vi "Alarm & Event List.vi"(8 "error in (no error)":errorcluster, 10 "Subview Stop Event":refnum<user-event>, 11 "Subsystem URL":refnum<k21>="\\\\localhost\\ABCDEFG\\TCU3") -> ()   [LabVIEW 2024]
doc: "Displays the current alarms and events for the specified subsystem. This VI is a subview of the Detailed View."
uses:
  Controls/Client/Alarm Description Item.ctl
  Controls/Client/Alarm & Event List - Data.ctl
  Controls/Client/Initialization Status.ctl
  <vilib>/lvdsc/alarm/Acknowledge Alarms By Instance.vi
  Shared/User Event - Stop.lvlib
  <vilib>/lvdsc/NI_DSC.lvlib
panel:
  out "error out":errorcluster
  in  "Acknowledge All":bool
  in  "Acknowledge":bool
  in  "Alarm Summary":i32(listbox)
  in  "Alarm Display Format":T1[](array[typedef])=[enum."alarm URL", enum."event?", enum."value", enum."set time", enum."ack time"]
  in  "Stop":bool
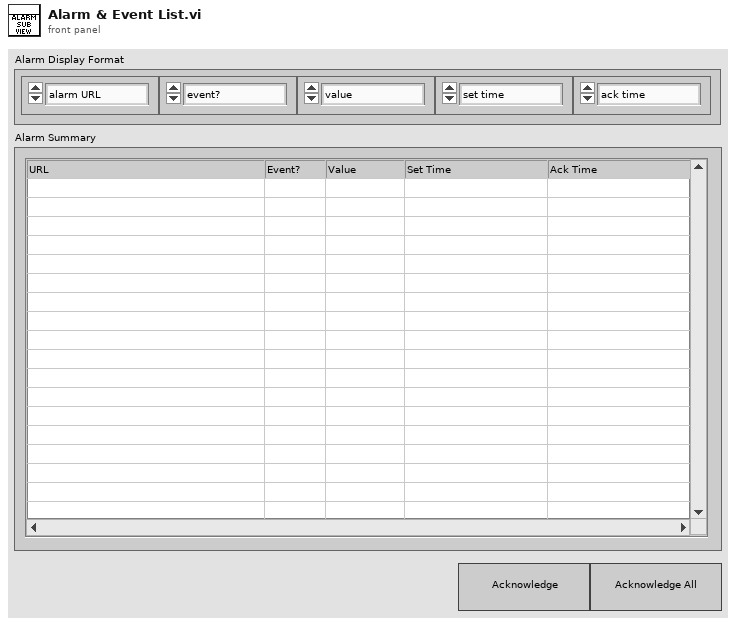
[diagram p1: front panel]
types:
  T1 = typedef "Alarm Description Item.ctl" = enum16{"alarm URL", "event?", "set time", "ack time", "clear time", "set user", "ack user", "clear user", "set point", "value", "priority", "alarm area", "alarm description", "ack comment"}
  T2 = typedef "Alarm & Event List - Data.ctl" = cluster{"Subsystem URL":refnum<k21>, "Variables":refnum<k21>[], "Subview Stop Event":refnum<user-event>, "Alarm & Event Notifications":refnum<user-event>, "Initialization Status":T3, "Value List Reference":refnum<vi>, "Alarms":cluster{"alarm URL":string, "set time":timestamp, "set user":string, "ack time":timestamp, "ack user":string, "clear time":timestamp, "clear user":string, "setpoint":enum16{""}, "value":dbl, "priority":u32, "alarm area":string, "alarm description":string, "ack comment":string, "event?":bool, "Refnum":u64}[]}
  T3 = typedef "Initialization Status.ctl" = enum16{"Initializing", "Initialized"}
  T4 = cluster{"alarm URL":string, "set time":timestamp, "set user":string, "ack time":timestamp, "ack user":string, "clear time":timestamp, "clear user":string, "setpoint":enum16{""}, "value":dbl, "priority":u32, "alarm area":string, "alarm description":string, "ack comment":string, "event?":bool, "Refnum":u64}
  T5 = cluster{"alarm URL":string, "set time":timestamp, "set user":string, "ack time":timestamp, "ack user":string, "clear time":timestamp, "clear user":string, "setpoint":enum16{""}, "value":dbl, "priority":u32, "alarm area":string, "alarm description":string, "ack comment":string, "event?":bool, "Refnum":u64}[]
  T6 = cluster{"alarm URL":string, "set time":timestamp, "set user":string, "ack time":timestamp, "ack user":string, "clear time":timestamp, "clear user":string, "setpoint":dbl, "value":dbl, "priority":u32, "alarm area":string, "alarm description":string, "ack comment":string, "event?":bool, "Refnum":u64}[]
  T7 = cluster{"# active alarms occurrences":i32, "any alarm occurrences?":bool, "# unack alarms occurrences":i32, "any unack alarm occurrences?":bool, "# shared variables with active alarms":i32, "any shared variables with alarms?":bool, "# shared variables with unack alarms":i32, "any shared variables with unack alarms?":bool}
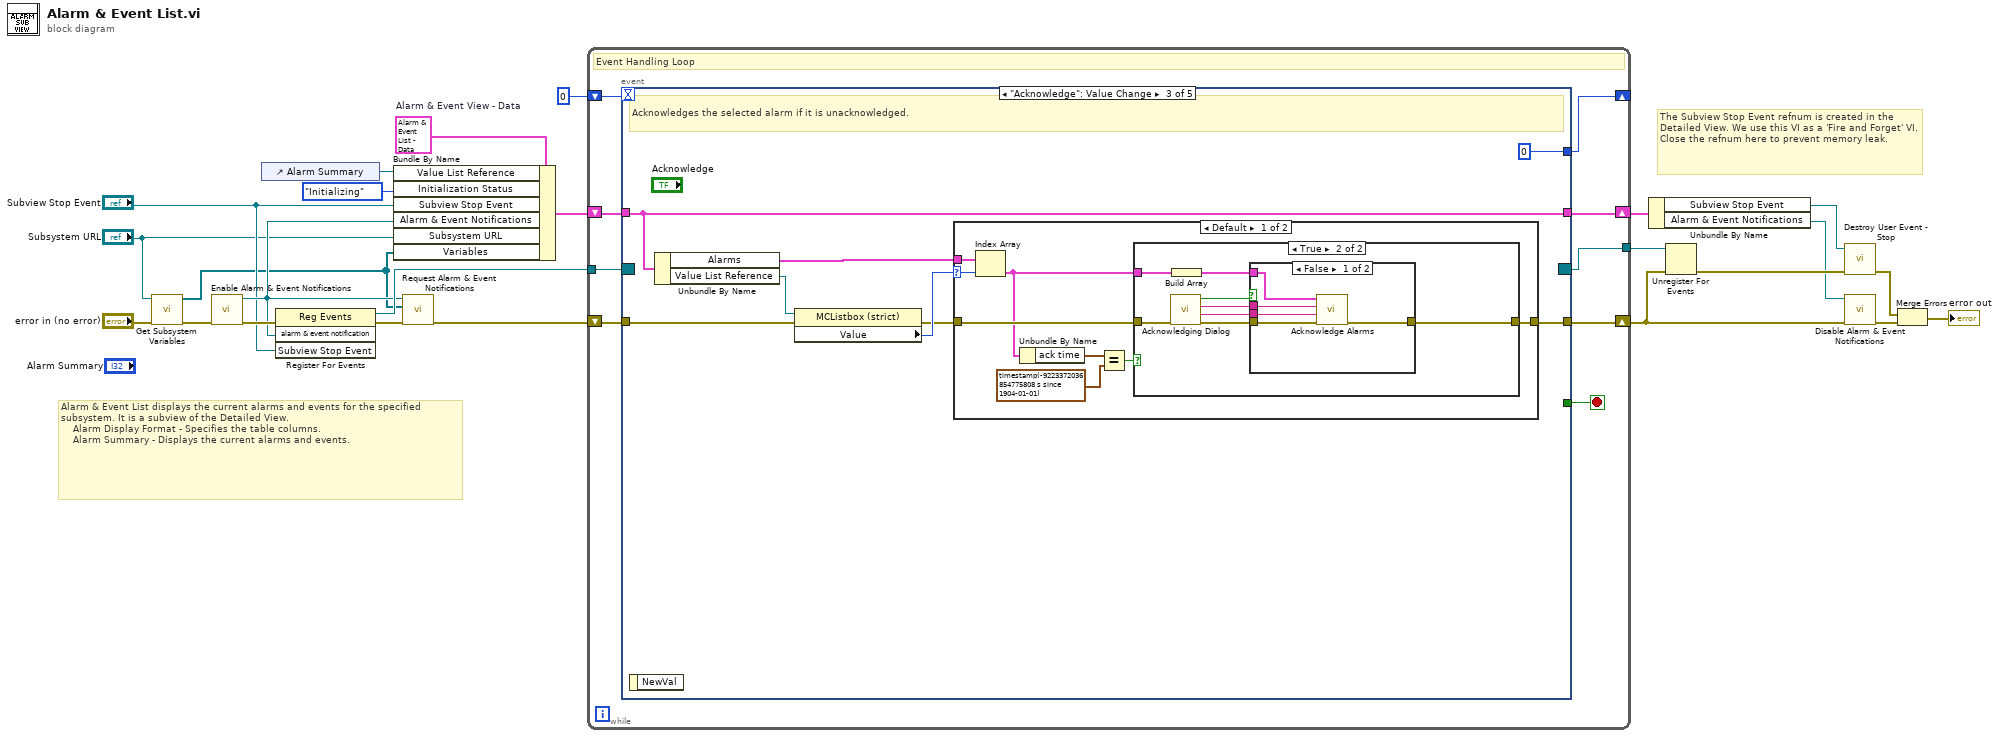
[diagram p0: block diagram]
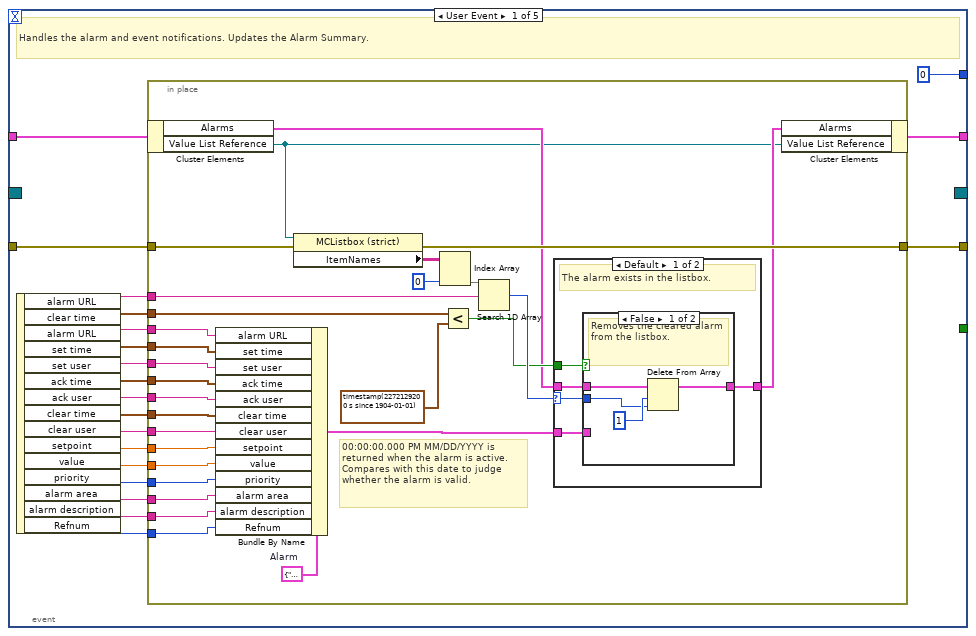
[diagram p2: hidden frame]
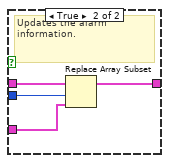
[diagram p3: hidden frame]
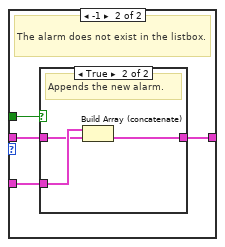
[diagram p4: hidden frame]
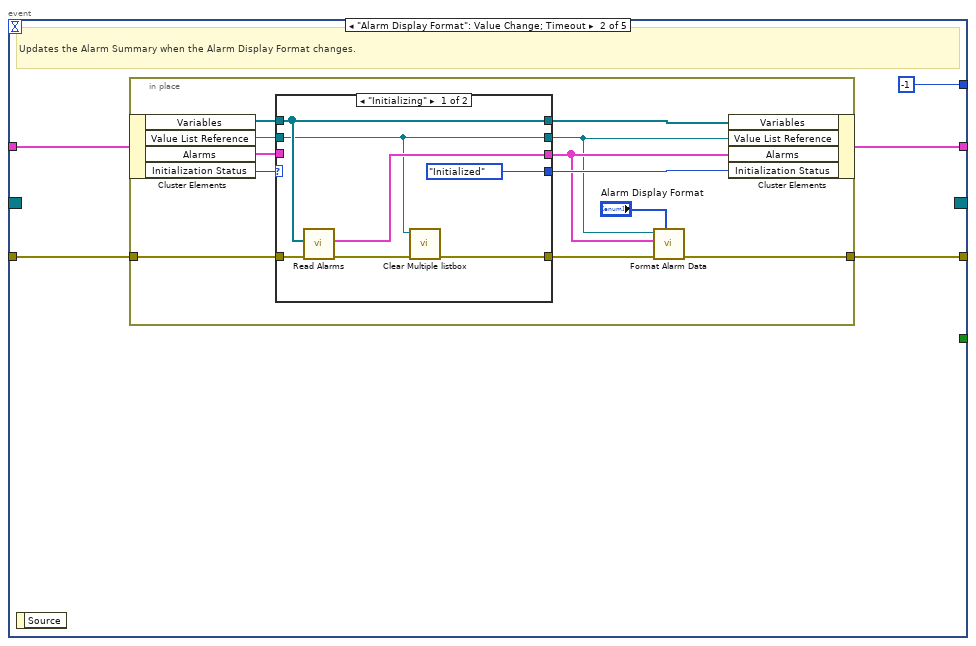
[diagram p6: hidden frame]
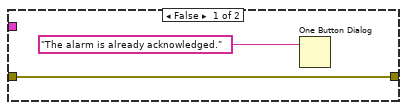
[diagram p8: hidden frame]
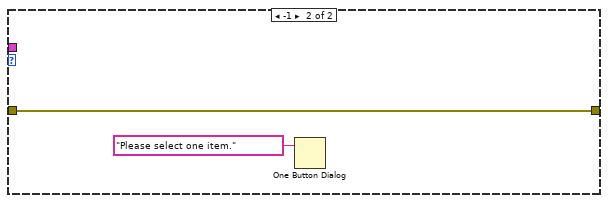
[diagram p10: hidden frame]
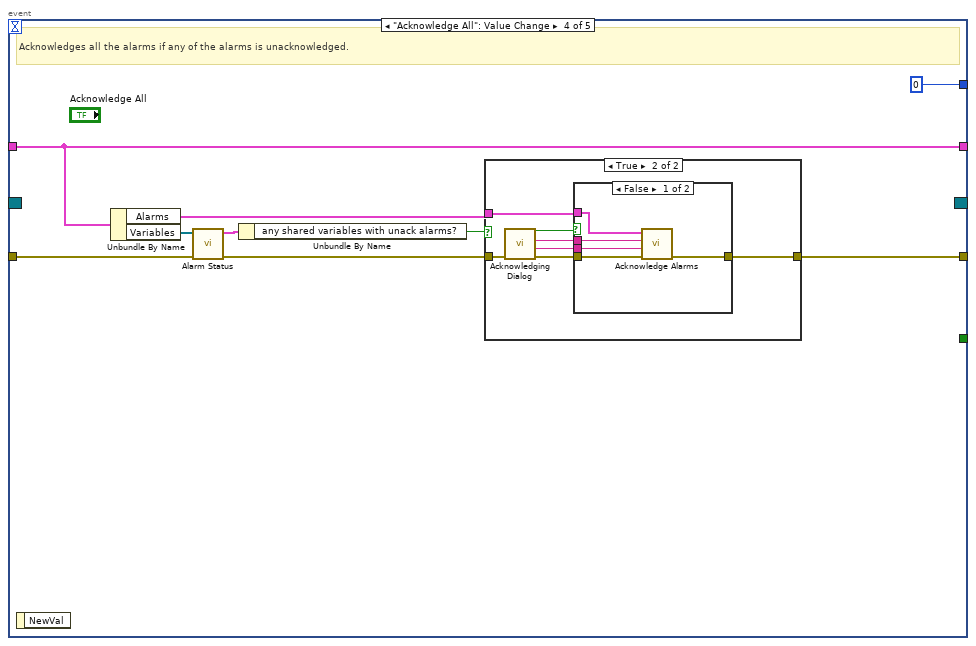
[diagram p11: hidden frame]
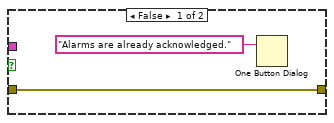
[diagram p12: hidden frame]
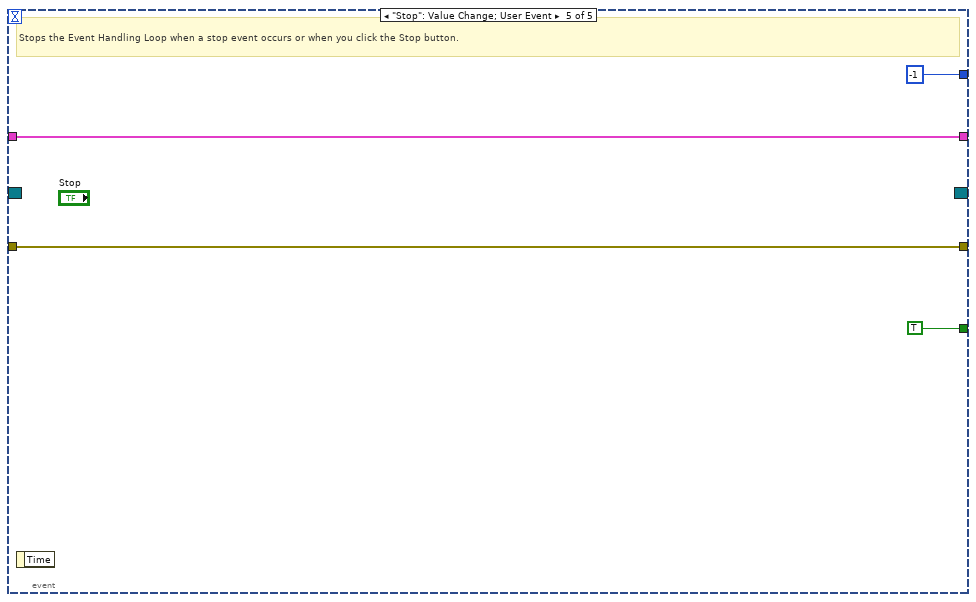
[diagram p14: hidden frame]
diagram:
  w14 = T2 {"Subsystem URL"="", "Variables"=[], "Subview Stop Event"=refnum, "Alarm & Event Notifications"=refnum, "Initialization Status"=enum."Initializing", "Value List Reference"=refnum, "Alarms"=[]}  # Alarm & Event View - Data
  # "The Subview Stop Event refnum is created in the Detailed View. We use this VI as a 'Fire and Forget' VI. Close the refnum here to prevent memory leak."
  # "Alarm & Event List displays the current alarms and events for the specified subsystem. It is a subview of the Detailed View.\n    Alarm Display Format - Specifies the table columns.\n    Alarm Summary - Displays the current alarms and events."
  n1 = call "Get Subsystem Variables.vi"("error in (no error)"="error in (no error)", "Subsystem URL"="Subsystem URL") -> ("error out"=w9:errorcluster, "Variable URLs"=w8:refnum<k21>[])  [unwired: 6 in, 2 out]
  n2 = call <vilib>:"Enable Alarm & Event Notifications.vi"("error in (no error)"=w9) -> ("error out"=w22:errorcluster, "alarm & event notification"=w13:refnum<user-event>)  [unwired: 9 out]
  n3 = control-ref of="Alarm Summary"() -> (w6:refnum<vi>)
  n4 = register-events(error in=w22, w13, "Subview Stop Event") -> (reference out=w21:refnum<event-registration>, error out=w23:errorcluster)  [unwired: 1 in]
  n5 = Bundle By Name(cluster=w14, "Value List Reference"=w6, "Initialization Status"=enum16{"Initializing", "Initialized"}."Initializing", "Subview Stop Event"="Subview Stop Event", "Alarm & Event Notifications"=w13, "Subsystem URL"="Subsystem URL", "Variables"=w8) -> (w11:T2)
  n6 = call <vilib>:"Request Alarm & Event Notifications.vi"("error in (no error)"=w23, "shared variables"=w8, "notification refnum"=w13) -> ("error out"=w20:errorcluster)  [unwired: 8 out]
  n7 = while {
    shift-right: [w30] -> w17
    shift-left: w20 -> [w31]
    tunnel: w21 -> [w32]
    tunnel: [w29] -> w24
    shift-right: [w25] -> w5
    shift-left: w11 -> [w28]
    shift-right: [w26] -> _
    shift-left: 0 -> [w27]
    stop <- w33 stop-if-true
    # "Event Handling Loop"
    n8 = event shown="[2] \"Acknowledge\": Value Change" {
      selector: w32 -> [_ _ _ _ _]
      dyn-events: [_ _ _ _ _] -> w29
      timeout: w27 -> [_ _ _ _ _]
      tunnel: [_ _ _ _ TRUE] -> w33
      tunnel: w31 -> [w40 w104 w138 w169 w191]
      tunnel: [w36 w103 w135 w174 w191] -> w30
      tunnel: w28 -> [w35 w106 w134 w172 w190]
      tunnel: [0 -1 0 0 -1] -> w26
      tunnel: [w34 w105 w134 w172 w190] -> w25
      event User Event {
        # "Handles the alarm and event notifications. Updates the Alarm Summary."
        n9 = event-data() -> ("alarm URL"=w39:string, "clear time"=w38:timestamp, "alarm URL"=w53:string, "set time"=w52:timestamp, "set user"=w51:string, "ack time"=w50:timestamp, "ack user"=w49:string, "clear time"=w48:timestamp, "clear user"=w47:string, "setpoint"=w46:dbl, "value"=w45:dbl, "priority"=w44:u32, "alarm area"=w43:string, "alarm description"=w42:string, "Refnum"=w41:u64)  [unwired: 1 in]
        n10 = in-place {
          in-place-border: w53 -> [w73]
          in-place-border: w52 -> [w72]
          in-place-border: w51 -> [w71]
          in-place-border: w50 -> [w70]
          in-place-border: w49 -> [w69]
          in-place-border: w48 -> [w68]
          in-place-border: w47 -> [w67]
          in-place-border: w46 -> [w66]
          in-place-border: w45 -> [w65]
          in-place-border: w44 -> [w64]
          in-place-border: w43 -> [w63]
          in-place-border: w42 -> [w62]
          in-place-border: w41 -> [w61]
          in-place-border: w40 -> [w60]
          in-place-border: w39 -> [w59]
          in-place-border: w38 -> [w58]
          in-place-border: [w57] -> w36
          w75 = T4 {"alarm URL"="", "set time"=timestamp(0 s since 1904-01-01), "set user"="", "ack time"=timestamp(0 s since 1904-01-01), "ack user"="", "clear time"=timestamp(0 s since 1904-01-01), "clear user"="", "setpoint"=enum."", "value"=0.0, "priority"=0, "alarm area"="", "alarm description"="", "ack comment"="", "event?"=FALSE, "Refnum"=0}  # Alarm
          # "00:00:00.000 PM MM/DD/YYYY is returned when the alarm is active. Compares with this date to judge whether the alarm is valid."
          n11 = in-place-cluster #1(w35) -> ("Alarms"=w56:T5, "Value List Reference"=w54:refnum<vi>)
          n12 = Bundle By Name(cluster=w75, "alarm URL"=w73, "set time"=w72, "set user"=w71, "ack time"=w70, "ack user"=w69, "clear time"=w68, "clear user"=w67, "setpoint"=w66, "value"=w65, "priority"=w64, "alarm area"=w63, "alarm description"=w62, "Refnum"=w61) -> (w78:T4)
          n13 = property class="MCListbox (strict)"(reference=w54, error in=w60) -> (error out=w57:errorcluster, "ItemNames"=w77:string[][])  [unwired: 1 out]
          n14 = Index Array(array=w77, index (col)=0 ("disabled index (col)")) -> (element=w80:string[])  [unwired: 1 in]
          n15 = Less?(x=w58, y=timestamp(2272129200 s since 1904-01-01)) -> (x < y?=w76:bool)
          n16 = Search 1D Array(1D array=w80, element=w59) -> (index of element=w79:i32)  [unwired: 1 in]
          n17 = case shown="Default" w79 {
            selector: w79 -> [w86 _]
            tunnel: [w84 w98] -> w55
            tunnel: w78 -> [w85 w97]
            tunnel: w76 -> [w83 w96]
            tunnel: w56 -> [w82 w95]
            frame Default {
              # "The alarm exists in the listbox."
              n18 = case shown="False" w83 {
                tunnel: w86 -> [w89 w94]
                tunnel: w85 -> [_ w93]
                tunnel: [w87 w92] -> w84
                tunnel: w82 -> [w88 w91]
                frame False {
                  # "Removes the cleared alarm from the listbox."
                  n19 = Delete From Array(array=w88, length=1 ("index"), index=w89) -> (array with subset deleted=w87:T5)  [unwired: 1 out]
                }
                frame True {
                  # "Updates the alarm information."
                  n20 = Replace Array Subset(array=w91, new element=w93, index=w94) -> (w92:T5)
                }
              }
            }
            frame -1 {
              # "The alarm does not exist in the listbox."
              n21 = case shown="True" w96 {
                tunnel: [w99 w102] -> w98
                tunnel: w97 -> [_ w101]
                tunnel: w95 -> [w99 w100]
                frame False {
                }
                frame True {
                  # "Appends the new alarm."
                  n22 = Build Array (concatenate)(w101, w100) -> (w102:T5)
                }
              }
            }
          }
          n23 = in-place-cluster #1("Alarms"=w55, "Value List Reference"=w54) -> (w34:T2)
        }
      }
      event "Alarm Display Format": Value Change; Timeout {
        # "Updates the Alarm Summary when the Alarm Display Format changes."
        n24 = event-data() -> ()  [unwired: 1 in, 1 out]
        n25 = in-place {
          in-place-border: [w109] -> w103
          in-place-border: w104 -> [w108]
          n26 = in-place-cluster #2(w106) -> ("Variables"=w119:refnum<k21>[], "Value List Reference"=w117:refnum<vi>, "Alarms"=w115:T5, "Initialization Status"=w118:T3)
          n27 = case shown="\"Initializing\"" w118 {
            selector: w118 -> [_ w129]
            tunnel: [w126 w131] -> w111
            tunnel: w117 -> [w122 w128]
            tunnel: w119 -> [w124 w130]
            tunnel: [w124 w130] -> w116
            tunnel: [w122 w128] -> w110
            tunnel: w115 -> [_ w131]
            tunnel: [enum16{"Initializing", "Initialized"}."Initialized" ("Initialization Status") w129] -> w113
            tunnel: [w121 w127] -> w112
            tunnel: w108 -> [w120 w127]
            frame "Initializing" {
              n28 = call <vilib>:"Read Alarms.vi"("error in (no error)"=w120, "shared variables"=w124) -> ("error out"=w125:errorcluster, "alarms"=w126:T6)  [unwired: 1 in, 7 out]
              n29 = call "Clear Multiple listbox.vi"("error in (no error)"=w125, "Listbox Reference In"=w122) -> ("error out"=w121:errorcluster)  [unwired: 8 in, 1 out]
            }
            frame "Initialized" {
            }
          }
          n30 = call "Format Alarm Data.vi"("Alarm Display Format"="Alarm Display Format", "error in (no error)"=w112, "Alarm Instances"=w111, "Multicolumn Listbox"=w110) -> ("error out"=w109:errorcluster)  [unwired: 1 in, 6 out]
          n31 = in-place-cluster #2("Variables"=w116, "Value List Reference"=w110, "Alarms"=w111, "Initialization Status"=w113) -> (w105:T2)
        }
      }
      event "Acknowledge": Value Change {
        # "Acknowledges the selected alarm if it is unacknowledged."
        n32 = event-data() -> ()  [unwired: 1 in, 1 out]
        n33 = Unbundle By Name(w134) -> ("Alarms"=w133:T5, "Value List Reference"=w132:refnum<vi>)
        n34 = property on="Property Node" class="MCListbox (strict)"(reference=w132, error in=w138) -> (error out=w136:errorcluster, "Value"=w137:i32)  [unwired: 1 out]
        n35 = case shown="Default" w137 {
          selector: w137 -> [w145 _]
          tunnel: w136 -> [w147 w165]
          tunnel: [w146 w165] -> w135
          tunnel: w133 -> [w143 _]
          frame Default {
            # "Item is selected."
            n36 = Index Array(array=w143, index=w145) -> (element=w142:T4)
            n37 = Unbundle By Name(w142) -> ("ack time"=w141:timestamp)
            n38 = Equal?(x=w141, y=timestamp(-9223372036854775808 s since 1904-01-01) ("ack time")) -> (x = y?=w144:bool)
            n39 = case shown="True" w144 {
              tunnel: w147 -> [w149 w153]
              tunnel: [w149 w152] -> w146
              tunnel: w142 -> [_ w150]
              frame False {
                n40 = One Button Dialog(message="The alarm is already acknowledged.") -> ()  [unwired: 1 in, 1 out]
              }
              frame True {
                n41 = call "Acknowledging Dialog.vi"("error in (no error)"=w153) -> ("error out"=w155:errorcluster, "Comment Out"=w157:string, "User Out"=w156:string, "Cancelled?"=w154:bool)  [unwired: 7 in]
                n42 = Build Array(w150) -> (w151:T5)
                n43 = case shown="False" w154 {
                  tunnel: w155 -> [w162 w163]
                  tunnel: w156 -> [w161 _]
                  tunnel: w157 -> [w160 _]
                  tunnel: [w159 w163] -> w152
                  tunnel: w151 -> [w158 _]
                  frame False {
                    n44 = call-poly <vilib>:"Acknowledge Alarms.vi"("error in (no error)"=w162, "comment"=w160, "acknowledging user"=w161, "alarms"=w158) -> ("error out"=w159:errorcluster)  [unwired: 7 in]
                  }
                  frame True {
                  }
                }
              }
            }
          }
          frame -1 {
            # "Item is NOT selected."
            n45 = One Button Dialog(message="Please select one item.") -> ()  [unwired: 1 in, 1 out]
          }
        }
      }
      event "Acknowledge All": Value Change {
        # "Acknowledges all the alarms if any of the alarms is unacknowledged."
        n46 = event-data() -> ()  [unwired: 1 in, 1 out]
        n47 = Unbundle By Name(w172) -> ("Alarms"=w171:T5, "Variables"=w167:refnum<k21>[])
        n48 = call <vilib>:"Alarm Status.vi"("error in (no error)"=w169, "shared variables"=w167) -> ("error out"=w168:errorcluster, "alarm summary data"=w170:T7)  [unwired: 8 in]
        n49 = Unbundle By Name(w170) -> ("any shared variables with unack alarms?"=w166:bool)
        n50 = case shown="True" w166 {
          tunnel: w168 -> [w176 w182]
          tunnel: [w176 w178] -> w174
          tunnel: w171 -> [_ w177]
          frame False {
            n51 = One Button Dialog(message="Alarms are already acknowledged.") -> ()  [unwired: 1 in, 1 out]
          }
          frame True {
            n52 = call "Acknowledging Dialog.vi"("error in (no error)"=w182) -> ("error out"=w181:errorcluster, "Comment Out"=w179:string, "User Out"=w180:string, "Cancelled?"=w183:bool)  [unwired: 7 in]
            n53 = case shown="False" w183 {
              tunnel: w177 -> [w184 _]
              tunnel: w181 -> [w188 w189]
              tunnel: w180 -> [w187 _]
              tunnel: w179 -> [w186 _]
              tunnel: [w185 w189] -> w178
              frame False {
                n54 = call-poly <vilib>:"Acknowledge Alarms.vi"("error in (no error)"=w188, "comment"=w186, "acknowledging user"=w187, "alarms"=w184) -> ("error out"=w185:errorcluster)  [unwired: 7 in]
              }
              frame True {
              }
            }
          }
        }
      }
      event "Stop": Value Change; User Event {
        # "Stops the Event Handling Loop when a stop event occurs or when you click the Stop button."
        n55 = event-data() -> ()  [unwired: 1 in, 1 out]
      }
    }
  }
  n56 = Unbundle By Name(w5) -> ("Subview Stop Event"=w3:refnum<user-event>, "Alarm & Event Notifications"=w4:refnum<user-event>)
  n57 = Unregister For Events(event registration refnum=w24, error in=w17) -> (error out=w15:errorcluster)
  n58 = call "Destroy User Event - Stop.vi"("error in (no error)"=w15, "User Event - Stop"=w3) -> ("error out"=w16:errorcluster)  [unwired: 9 in]
  n59 = call <vilib>:"Disable Alarm & Event Notifications.vi"("error in (no error)"=w17, "notification refnum"=w4) -> ("error out"=w19:errorcluster)  [unwired: 9 out]
  n60 = Merge Errors(w16, w19) -> (→"error out":errorcluster)
